vi "EmergencyGLOBAL (1).vi"() -> ()   [LabVIEW 2017]
panel:
  in  "Manifold Temperature Range":dbl[](array[numeric])=[60.0, -60.0]
  in  "IMU Temperature":dbl[](array[numeric])=[85.0, -20.0]
  in  "Tank Temperature Range":dbl[](array[numeric])=[60.0, -50.0]
  in  "Battery Temperature Range":dbl[](array[numeric])=[50.0, -10.0]
  in  "Compact RIO Temperature Range":dbl[](array[numeric])=[80.0, -15.0]
  in  "Battery Voltage":dbl=20.0
  in  "Hall Effect":dbl=0.1
  in  "HPPT":dbl=-1000.0
  in  "PT":dbl=-30.0
  # "-60 - 0 -> disconnected"
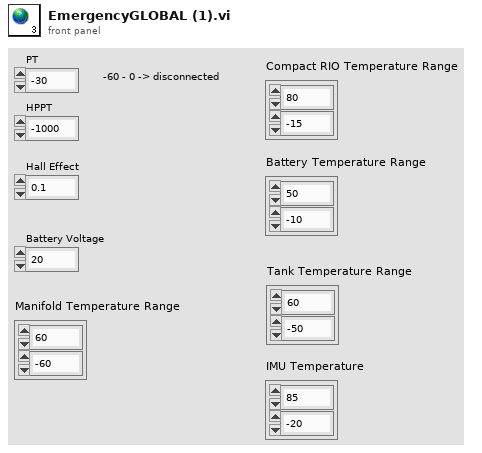
[diagram p1: front panel]
diagram:
